vi "Hello World.vi"(10 "String":string, 11 "Hello World in":refnum<class "Hello World.lvclass">) -> (3 "Hello World out":refnum<class "Hello World.lvclass">)   [LabVIEW 2021, in "Hello World Event.lvlib" / "Hello World Msg Strategy.lvlib" / "Hello World.lvclass"]
uses:
  Hello World.lvclass
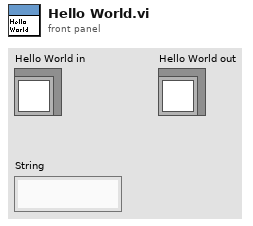
[diagram p1: front panel]
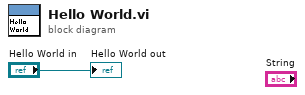
[diagram p0: block diagram]
diagram:
  "Hello World out" <- "Hello World in"
